vi "Master.vi"   [LabVIEW 2016, in "Moving Motor.lvrbt"]
uses:
  Moving Motor.lvrbt
  <vilib>/NXT/Block Support/NXT_InputPort.ctl
  <vilib>/NXT/Hardware/Plugins/Tetrix DC Motor/TetrixDCMotorAddress.ctl
  <vilib>/NXT/NXTIO Xnodes/NXTIONodeSubVIs/TETRIX IO Move DC Motors.vi
  <vilib>/NXT/Dual Mode Library/Sensors/EV3_Color_Color.vi
  <vilib>/NXT/NXTIO Xnodes/NXTIONodeSubVIs/TETRIX IO Stop DC Motors.vi
  <vilib>/NXT/Dual Mode Library/Waits/Wait_Num.vi
  <vilib>/NXT/Subs/LVHSConnector.ctl
  <vilib>/NXT/NXTIO Xnodes/AddressXNode/NXTIOAddress.xnode
  <vilib>/NXT/NXTIO Xnodes/NXTIOXNode/NXTIO.xnode
  <vilib>/NXT/LegoClasses/BrickReference/BrickReference.lvclass
types:
  T1 = typedef "TetrixDCMotorAddress.ctl" = i32
  T2 = typedef "LVHSConnector.ctl" = refnum<class "BrickReference.lvclass">
  T3 = cluster{"TetrixDCMotor":T1, "TetrixDCMotor 2":T1}
  T4 = typedef "NXT_InputPort.ctl" = u32
  T5 = typedef "ColorSensorColors.ctl" = enum16{"No Color", "Black", "Blue", "Green", "Yellow", "Red", "White", "Brown"}
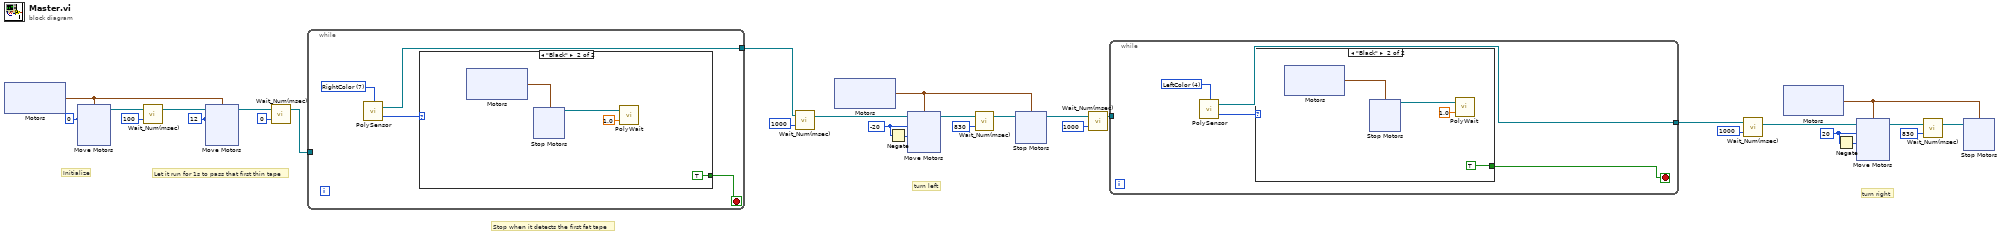
[diagram p0: block diagram]
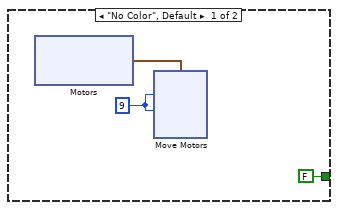
[diagram p2: hidden frame]
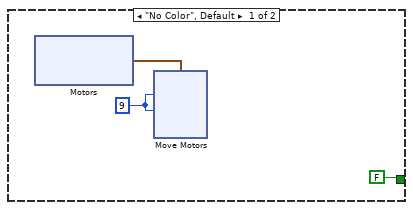
[diagram p3: hidden frame]
diagram:
  w6 = i8 20 ("Power/Speed 1")
  w17 = i8 -20 ("Power/Speed 1")
  w14 = i8 12 ("Power/Speed 1")
  w30 = i8 0 ("Power/Speed 1")
  # "turn right"
  # "turn left"
  # "Stop when it detects the first fat tape"
  # "Let it run for 1s to pass that first thin tape"
  # "Initialize"
  n1 = xnode "Motors"() -> ("Motor"=w24:cluster{"TetrixDCMotor":T1, "TetrixDCMotor":T1})
  n2 = xnode "Move Motors"("Power/Speed 2"=w30, "Power/Speed 1"=w30, "Motors"=w24) -> ("NXT/EV3"=w29:T2)  [unwired: 1 in]
  n3 = call <vilib>:"Wait_Num(msec).vi"("Time (100 msec)"=u32 100, "NXT/EV3"=w29) -> ("NXT/EV3"=w25:T2)  [unwired: 2 in]
  n4 = xnode "Move Motors"("Power/Speed 2"=w14, "Power/Speed 1"=w14, "Motors"=w24, "NXT/EV3"=w25) -> ("NXT/EV3"=w27:T2)
  n5 = call <vilib>:"Wait_Num(msec).vi"("Time (100 msec)"=u32 0, "NXT/EV3"=w27) -> ("NXT/EV3"=w23:T2)  [unwired: 2 in]
  n6 = while {
    tunnel: w23 -> [_]
    tunnel: [w31] -> w2
    stop <- w32 stop-if-true
    w34 = T4 7 items=["Port 1"=0, "Port 2"=1, "Port 3"=2, "Port 4"=3, "LeftColor"=4, "RightColor"=7] ("Port (Port 1)")
    n7 = call-poly <vilib>:"PolySensor.vi"("Port (Port 1)"=w34) -> ("Detected Color"=w33:T5, "NXT/EV3"=w31:T2)  [unwired: 2 in]
    n8 = case shown="\"Black\"" w33 {
      tunnel: [FALSE TRUE] -> w32
      frame "No Color", Default {
        w36 = i8 9 ("Power/Speed 1")
        n9 = xnode "Motors"() -> ("Motor"=w37:cluster{"TetrixDCMotor":T1, "TetrixDCMotor":T1})
        n10 = xnode "Move Motors"("Power/Speed 2"=w36, "Power/Speed 1"=w36, "Motors"=w37) -> ()  [unwired: 1 in, 1 out]
      }
      frame "Black" {
        n11 = xnode "Motors"() -> ("Motor"=w50:cluster{"TetrixDCMotor":T1, "TetrixDCMotor":T1})
        n12 = xnode "Stop Motors"("Motors"=w50) -> ("NXT/EV3"=w48:T2)  [unwired: 1 in]
        n13 = call-poly <vilib>:"PolyWait.vi"("Time (1 sec)"=sgl 1.0, "NXT/EV3"=w48) -> ()  [unwired: 2 in, 1 out]
      }
    }
  }
  n14 = call <vilib>:"Wait_Num(msec).vi"("Time (100 msec)"=u32 1000, "NXT/EV3"=w2) -> ("NXT/EV3"=w15:T2)  [unwired: 2 in]
  n15 = xnode "Motors"() -> ("Motor"=w19:cluster{"TetrixDCMotor":T1, "TetrixDCMotor":T1})
  n16 = Negate(x=w17) -> (-x=w18:i8)
  n17 = xnode "Move Motors"("Power/Speed 2"=w18, "Power/Speed 1"=w17, "Motors"=w19, "NXT/EV3"=w15) -> ("NXT/EV3"=w22:T2)
  n18 = call <vilib>:"Wait_Num(msec).vi"("Time (100 msec)"=u32 830, "NXT/EV3"=w22) -> ("NXT/EV3"=w20:T2)  [unwired: 2 in]
  n19 = xnode "Stop Motors"("Motors"=w19, "NXT/EV3"=w20) -> ("NXT/EV3"=w12:T2)
  n20 = call <vilib>:"Wait_Num(msec).vi"("Time (100 msec)"=u32 1000, "NXT/EV3"=w12) -> ("NXT/EV3"=w3:T2)  [unwired: 2 in]
  n21 = while {
    tunnel: w3 -> [_]
    tunnel: [w58] -> w1
    stop <- w57 stop-if-true
    w60 = T4 4 items=["Port 1"=0, "Port 2"=1, "Port 3"=2, "Port 4"=3, "LeftColor"=4, "RightColor"=7] ("Port (Port 1)")
    n22 = call-poly <vilib>:"PolySensor.vi"("Port (Port 1)"=w60) -> ("Detected Color"=w59:T5, "NXT/EV3"=w58:T2)  [unwired: 2 in]
    n23 = case shown="\"Black\"" w59 {
      tunnel: [FALSE TRUE] -> w57
      frame "No Color", Default {
        w62 = i8 9 ("Power/Speed 1")
        n24 = xnode "Motors"() -> ("Motor"=w63:cluster{"TetrixDCMotor":T1, "TetrixDCMotor":T1})
        n25 = xnode "Move Motors"("Power/Speed 2"=w62, "Power/Speed 1"=w62, "Motors"=w63) -> ()  [unwired: 1 in, 1 out]
      }
      frame "Black" {
        n26 = xnode "Motors"() -> ("Motor"=w76:cluster{"TetrixDCMotor":T1, "TetrixDCMotor":T1})
        n27 = xnode "Stop Motors"("Motors"=w76) -> ("NXT/EV3"=w74:T2)  [unwired: 1 in]
        n28 = call-poly <vilib>:"PolyWait.vi"("Time (1 sec)"=sgl 1.0, "NXT/EV3"=w74) -> ()  [unwired: 2 in, 1 out]
      }
    }
  }
  n29 = call <vilib>:"Wait_Num(msec).vi"("Time (100 msec)"=u32 1000, "NXT/EV3"=w1) -> ("NXT/EV3"=w4:T2)  [unwired: 2 in]
  n30 = xnode "Motors"() -> ("Motor"=w8:cluster{"TetrixDCMotor":T1, "TetrixDCMotor":T1})
  n31 = Negate(x=w6) -> (-x=w7:i8)
  n32 = xnode "Move Motors"("Power/Speed 2"=w7, "Power/Speed 1"=w6, "Motors"=w8, "NXT/EV3"=w4) -> ("NXT/EV3"=w11:T2)
  n33 = call <vilib>:"Wait_Num(msec).vi"("Time (100 msec)"=u32 830, "NXT/EV3"=w11) -> ("NXT/EV3"=w9:T2)  [unwired: 2 in]
  n34 = xnode "Stop Motors"("Motors"=w8, "NXT/EV3"=w9) -> ()  [unwired: 1 out]
